vi "Get Test File Path.vi"(10 "Test Name":string, 11 "Folder Name":string) -> (3 "test path":path)   [LabVIEW 2020, in "Settings.lvlib"]
uses:
  Settings.lvlib
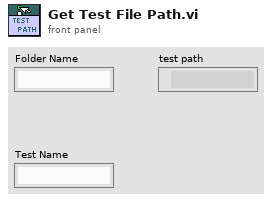
[diagram p1: front panel]
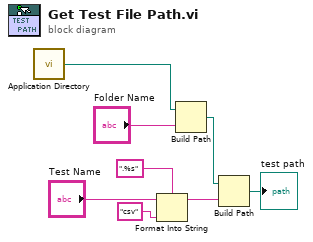
[diagram p0: block diagram]
diagram:
  n1 = call <vilib>:"Application Directory.vi"() -> ("Application Directory"=w1:path)
  n2 = Format Into String(format string=".%s", initial string="Test Name", "csv" ("format string")) -> (resulting string=w3:string)  [unwired: 1 in, 1 out]
  n3 = Build Path(base path=w1, name or relative path="Folder Name") -> (appended path=w2:path)
  n4 = Build Path(base path=w2, name or relative path=w3) -> (appended path=→"test path":path)
